vi "Object_Track_Webcam_PC.vi"() -> ()   [LabVIEW 2017]
doc: "This example demonstrates the Traditional MeanShift algorithm to track an object in the image."
uses:
  <vilib>/userdefined/High Color/IMAQdx.ctl
  <vilib>/vision/driver/NI_Vision_Acquisition_Software.lvlib
panel:
  out "Distance":dbl
  in  "Stop":bool
  out "Image":T1(plugin-control)
  # "Overview: Demonstrate the Traditional MeanShift algorithm to track an object in the image.\nRequirements: LabVIEW Full Development System and Vision Development Module.\nInstructions: Run the VI."
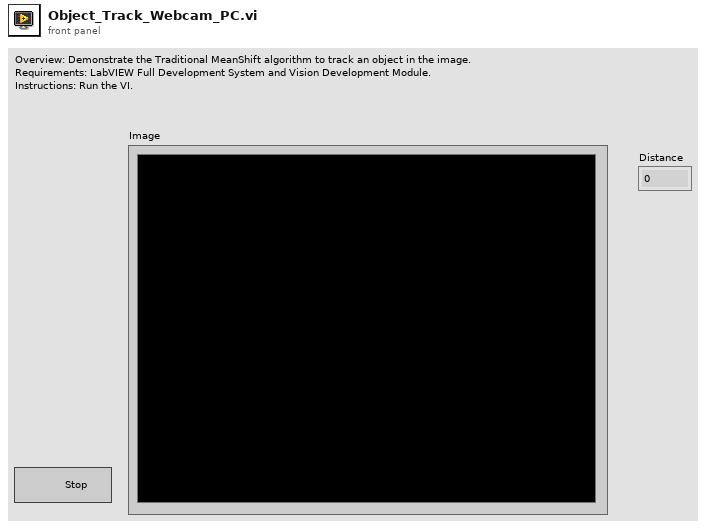
[diagram p1: front panel]
types:
  T1 = typedef "IMAQ Image.ctl" = refnum<image>
  T2 = typedef "IMAQdx.ctl" = refnum<k21>
  T3 = typedef "Image Type" = u32
  T4 = cluster{"Number of Histogram Bins":i32, "Blending Parameter (%)":dbl, "Maximum Iterations":i32}
  T5 = typedef "IMAQ Object Tracking Session.ctl" = refnum<k20>
  T6 = typedef "IMAQ Point" = cluster{"X":sgl, "Y":sgl}
  T7 = typedef "ROI Descriptor" = cluster{"Global Rectangle":i32[], "Contours":cluster{"ID":enum32{"External", "Internal"}, "Type":u32, "Coordinates":i32[]}[]}
  T8 = cluster{"Label":string, "Score":i32, "Angle":dbl, "Location":cluster{"X":dbl, "Y":dbl}, "Bounding Box":cluster{"X":dbl, "Y":dbl}[], "Object Found?":bool}[]
  T9 = cluster{"Label":string, "Score":i32, "Angle":dbl, "Location":cluster{"X":dbl, "Y":dbl}, "Bounding Box":cluster{"X":dbl, "Y":dbl}[], "Object Found?":bool}
  T10 = cluster{"Desired Font (Application)":enum16{"User-specified Font", "Application Font", "System Font", "Dialog Font"}, "[User-specified Font]":cluster{"Font Name":string, "Size":i16, "Strikeout?":bool, "Italic?":bool, "Underline?":bool, "Outline?":bool, "Shadow?":bool, "Bold?":bool, "Rotation Angle":dbl}, "Horizontal Alignment":i16, "Vertical Alignment":i16}
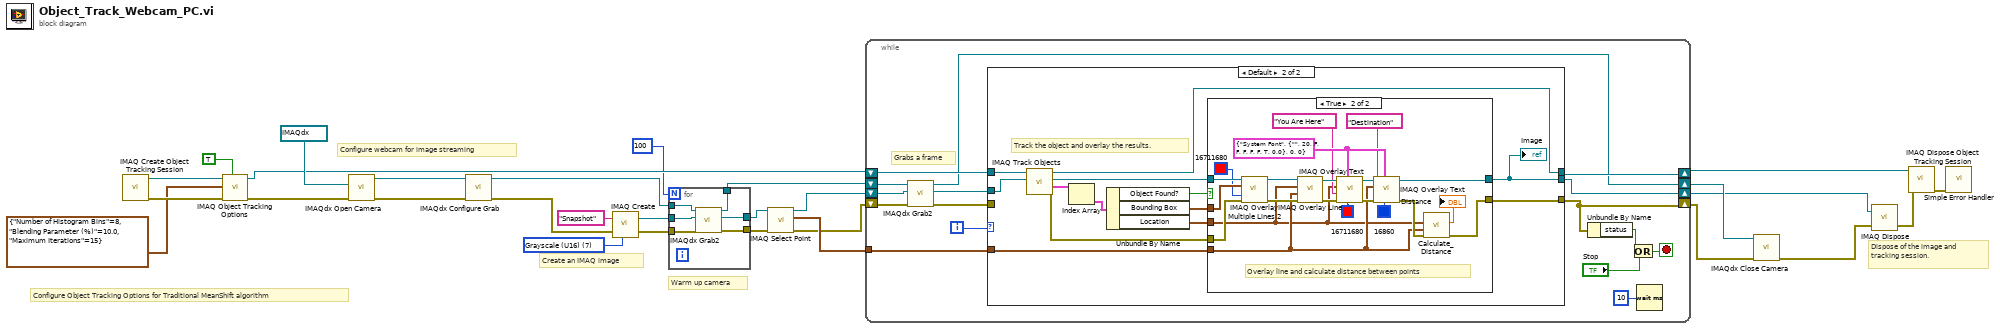
[diagram p0: block diagram]
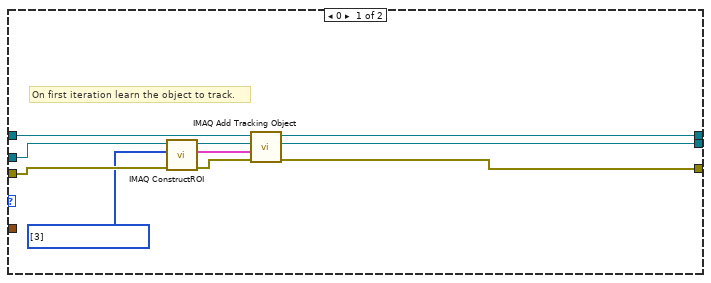
[diagram p2: hidden frame]
diagram:
  w21 = T3 7 items=["Grayscale (U8)", "Grayscale (I16)", "Grayscale (SGL)", "Complex (CSG)", "RGB (U32)", "HSL (U32)", "RGB (U64)", "Grayscale (U16)"] ("Image Type")
  # "Warm up camera"
  # "Create an IMAQ image"
  # "Configure webcam for image streaming"
  # "Configure Object Tracking Options for Traditional MeanShift algorithm"
  # "Dispose of the image and tracking session."
  n1 = call "IMAQ Create Object Tracking Session"() -> ("error out"=w24:errorcluster, "Object Tracking Session"=w26:T5)  [unwired: 1 in, 9 out]
  n2 = call-poly "IMAQ Object Tracking Options"("Get/Set (Get)"=TRUE, "error in (no error)"=w24, "Mean Shift Options in"=T4 {"Number of Histogram Bins"=8, "Blending Parameter (%)"=10.0, "Maximum Iterations"=15}, "Object Tracking Session In"=w26) -> ("error out"=w20:errorcluster, "Object Tracking Session Out"=w15:T5)  [unwired: 5 in, 1 out]
  n3 = call <vilib>:"IMAQdx Open Camera.vi"("error in"=w20, "Session In"=T2 "cam1") -> ("error out"=w17:errorcluster, "Session Out"=w18:T2)  [unwired: 8 in]
  n4 = call <vilib>:"IMAQdx Configure Grab.vi"("error in"=w17, "Session In"=w18) -> ("error out"=w14:errorcluster, "Session Out"=w10:T2)  [unwired: 8 in]
  n5 = call "IMAQ Create"("Image Name"="Snapshot", "Image Type"=w21, "error in (no error)"=w14) -> ("New Image"=w9:T1, "error out"=w8:errorcluster)  [unwired: 2 in]
  n6 = for {
    N: 100 -> [_]
    tunnel: w10 -> [w35]
    tunnel: w9 -> [w34]
    tunnel: w8 -> [w33]
    tunnel: [w32] -> w5
    tunnel: [w31] -> w4
    tunnel: [w30] -> w7
    n7 = call <vilib>:"IMAQdx Grab2.vi"("error in"=w33, "Image In"=w34, "Session In"=w35) -> ("error out"=w32:errorcluster, "Image Out"=w31:T1, "Session Out"=w30:T2)  [unwired: 5 in, 1 out]
  }
  n8 = call "IMAQ Select Point"("error in (no error)"=w5, "Image In"=w4) -> ("error out"=w1:errorcluster, "Point"=w3:T6, "Image Out (duplicate)"=w2:T1)  [unwired: 6 in, 1 out]
  n9 = while {
    shift-right: [w48] -> w29
    shift-left: w15 -> [w49]
    shift-right: [w44] -> w12
    shift-left: w1 -> [w45]
    shift-right: [w40] -> w13
    shift-left: w7 -> [w43]
    tunnel: w3 -> [w36]
    shift-right: [w50] -> w6
    shift-left: w2 -> [w37]
    i -> [w42]
    stop <- w46 stop-if-true
    # "Grabs a frame"
    n10 = call <vilib>:"IMAQdx Grab2.vi"("error in"=w45, "Image In"=w37, "Session In"=w43) -> ("error out"=w41:errorcluster, "Image Out"=w38:T1, "Session Out"=w40:T2)  [unwired: 5 in, 1 out]
    n11 = case shown="Default" w42 {
      tunnel: [w58 w74] -> w48
      tunnel: [w60 w64] -> w50
      tunnel: [w59 w65] -> w44
      tunnel: w49 -> [w61 w70]
      tunnel: w38 -> [w52 w66]
      tunnel: w41 -> [w55 _]
      tunnel: w36 -> [_ w62]
      frame 0 {
        w53 = u32[] [3] items=["No Selection", "Point", "Line", "Rectangle", "Oval", "Polygon", "Freehand Region", "Annulus", "Zoom", "Pan", "Broken Line", "Freehand Line", "Rotated Rectangle"] ("Tools")
        # "On first iteration learn the object to track."
        n12 = call "IMAQ ConstructROI"("error in (no error)"=w55, "Tools"=w53, "Image"=w52) -> ("error out"=w54:errorcluster, "ROI Descriptor Out"=w56:T7, "Image Out (duplicate)"=w57:T1)  [unwired: 5 in, 1 out]
        n13 = call "IMAQ Add Tracking Object"("error in (no error)"=w54, "ROI Descriptor"=w56, "Image"=w57, "Object Tracking Session In"=w61) -> ("error out"=w59:errorcluster, "Image (duplicate)"=w60:T1, "Object Tracking Session Out"=w58:T5)  [unwired: 1 in, 4 out]
      }
      frame Default {
        # "Track the object and overlay the results."
        n14 = call "IMAQ Track Objects"("Image"=w66, "Object Tracking Session In"=w70) -> ("error out"=w69:errorcluster, "Objects (pixel)"=w73:T8, "Image (duplicate)"=w72:T1, "Object Tracking Session Out"=w74:T5)  [unwired: 2 in, 4 out]
        n15 = Index Array(array=w73) -> (element=w68:T9)  [unwired: 1 in]
        n16 = Unbundle By Name(w68) -> ("Object Found?"=w67:bool, "Bounding Box"=w71:cluster{"X":dbl, "Y":dbl}[], "Location"=w63:cluster{"X":dbl, "Y":dbl})
        n17 = case shown="True" w67 {
          tunnel: w72 -> [w75 w97]
          tunnel: [w75 w79] -> w64
          tunnel: w71 -> [_ w95]
          tunnel: w69 -> [w76 w96]
          tunnel: [w76 w78] -> w65
          tunnel: w63 -> [_ w80]
          tunnel: w62 -> [_ w81]
          frame False {
          }
          frame True {
            w84 = T10 {"Desired Font (Application)"=enum."System Font", "[User-specified Font]"={"Font Name"="", "Size"=20, "Strikeout?"=FALSE, "Italic?"=FALSE, "Underline?"=FALSE, "Outline?"=FALSE, "Shadow?"=FALSE, "Bold?"=TRUE, "Rotation Angle"=0.0}, "Horizontal Alignment"=0, "Vertical Alignment"=0} ("Font, Size & Style")
            # "Overlay line and calculate distance between points"
            n18 = call "IMAQ Overlay Multiple Lines 2"("Image"=w97, "Line End Points"=w95, "Color"=u32 16711680, "error in (no error)"=w96) -> ("Image Out"=w92:T1, "error out"=w91:errorcluster)  [unwired: 4 in, 6 out]
            n19 = call "IMAQ Overlay Line"("error in (no error)"=w91, "End Point"=w81, "Start Point"=w80, "Image"=w92) -> ("error out"=w85:errorcluster, "Image Out"=w86:T1)  [unwired: 6 in]
            n20 = call "IMAQ Overlay Text"("Text Color (black)"=u32 16711680, "Font, Size & Style"=w84, "error in (no error)"=w85, "String"="You Are Here", "Origin"=w80, "Image"=w86) -> ("error out"=w88:errorcluster, "Image Out"=w87:T1)  [unwired: 4 in]
            n21 = call "IMAQ Overlay Text"("Text Color (black)"=u32 16860, "Font, Size & Style"=w84, "error in (no error)"=w88, "String"="Destination", "Origin"=w81, "Image"=w87) -> ("error out"=w82:errorcluster, "Image Out"=w79:T1)  [unwired: 4 in]
            n22 = call "Calculate_Distance.vi"("error in (no error)"=w82, "Destination"=w81, "Position"=w80) -> ("error out"=w78:errorcluster, "Distance"=→"Distance":dbl)  [unwired: 7 in]
          }
        }
        "Image" <- w64
      }
    }
    n23 = Unbundle By Name(w44) -> ("status"=w51:bool)
    n24 = Or(x=w51, y="Stop") -> (x .or. y?=w46:bool)
    n25 = Wait (ms)(milliseconds to wait=u32 10) -> ()  [unwired: 1 out]
  }
  n26 = call <vilib>:"IMAQdx Close Camera.vi"("error in"=w12, "Session In"=w13) -> ("error out"=w16:errorcluster)  [unwired: 9 in]
  n27 = call "IMAQ Dispose"("Image"=w6, "error in (no error)"=w16) -> ("error out"=w28:errorcluster)  [unwired: 1 in, 3 out]
  n28 = call "IMAQ Dispose Object Tracking Session"("error in (no error)"=w28, "Object Tracking Session"=w29) -> ("error out"=w27:errorcluster)  [unwired: 9 out]
  n29 = call <vilib>:"Simple Error Handler.vi"("error in (no error)"=w27) -> ()  [unwired: 1 in, 8 out]
